vi "NI VeriStand - Notify New Log Files Complete.vi"(8 "error in (no error)":errorcluster, 9 "timeout in ms (10000)":i32=10000, 10 "Log File Paths":path[](array[path]), 11 "Item Ref in":T1 format="%.0x") -> (0 "error out":errorcluster, 1 "timed out?":bool, 3 "Item Ref out":T1 format="%.0x")   [LabVIEW 2020, in "Custom Device API.lvlib"]
doc: "Sends a notification to clients connected through the VeriStand Gateway that the specified custom device item completed a new log file."
uses:
  <vilib>/NI VeriStand/Custom Device API/Custom Device API.lvlib
  <vilib>/NI VeriStand/Custom Device API/Custom Device Item Ref.ctl
  060c0dcc-2ffd-4d89-9872-407ac3d10f78.vi
  <vilib>/NI VeriStand/Custom Device API/Custom Device Offline Path.vi
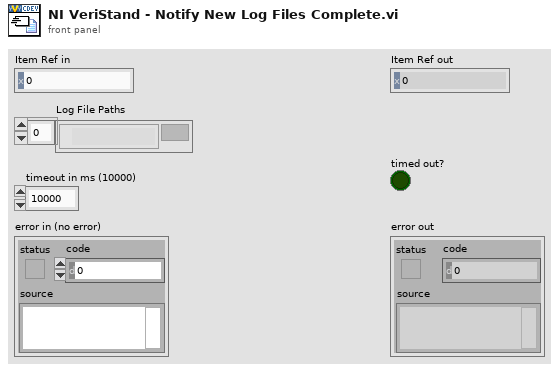
[diagram p1: front panel]
types:
  T1 = typedef "Custom Device API.lvlib/Custom Device Item Ref.ctl" = u64
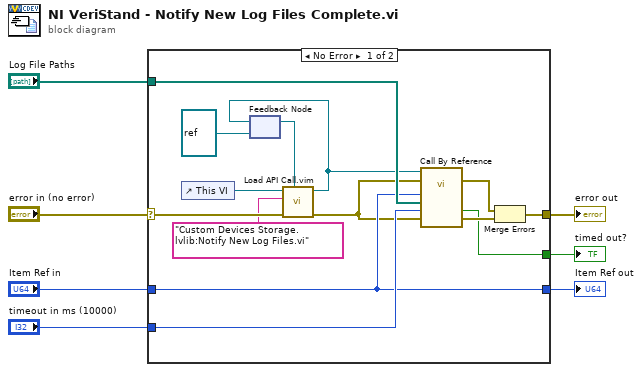
[diagram p0: block diagram]
diagram:
  n1 = case shown="No Error" "error in (no error)" {
    selector: "error in (no error)" -> [w13 w23]
    tunnel: [w20 w23] -> w7
    tunnel: "Item Ref in" -> [w16 w22]
    tunnel: [w16 w22] -> w5
    tunnel: "Log File Paths" -> [w19 _]
    tunnel: "timeout in ms (10000)" -> [w18 _]
    tunnel: [w17 _] -> w2
    frame No Error {
      n2 = control-ref of="This VI"() -> (w14:refnum<vi>)
      n3 = feedback #1(refnum<vi> refnum ("type specifier VI Refnum (for type only)")) -> (w15:refnum<vi>)
      n4 = call "Load API Call.vim"("VI reference in"=w15, "error in (no error)"=w13, "VI qualified name"="Custom Devices Storage.lvlib:Notify New Log Files.vi", "Caller VI ref"=w14) -> ("error out"=w12:errorcluster, "VI reference"=w11:refnum<vi>)  [unwired: 6 in]
      n5 = feedback-in #1(w11) -> ()
      n6 = call-by-ref "?"(reference=w11, error in=w12, 8:"error in (no error)"=w12, "timeout in ms (10000)"=w18, "Paths"=w19, "Item Ref"=w16) -> (error out=w8:errorcluster, 0:"error out"=w21:errorcluster, "timed out?"=w17:bool)  [unwired: 6 in, 1 out]
      n7 = Merge Errors(w8, w21) -> (w20:errorcluster)
    }
    frame Error {
    }
  }
  "Item Ref out" <- w5
  "error out" <- w7
  "timed out?" <- w2
